vi "Sub Super Duper_7_02a_JW.vi"(0 "VISA resource name":refnum<visa-resource-name>="GPIB0::17::INSTR", 1 "Sample Properties:":T5 {"Date Created" format="%<%Y/%m/%d>T"}, 2 "TRF Cluster":T6={"Step 4"=-38.0, "# of Loops"=1.0, "Transfer 2"=FALSE, "Start 4"=-2.0, "Total Points 2"=2, "Start 3"=40.0, "Stop 2"=-40.0, "Step 3"=-1.0, "Loop Step"=0.0, "Integration Time 3"=0, "Loop Wait"=0.0, "First Step"=0.0} {"Loop Wait" format="%<%H:%M:%S>t"; "Integration Time 3" scale=0.0..2.0; "Step 3" format="%.2f"; "Stop 2" format="%.2f"; "Start 3" format="%.2f"; "Start 4" format="%.2f"; "Step 4" format="%.2f"}, 3 "TSP Cluster":T7={"Transport"=FALSE, "Start 2"=0.0, "Stop 3"=-60.0, "Step 2"=-1.0, "Start"=0.0, "Step"=-10.0, "Total Points"=7, "Integration Time"=0} {"Integration Time" scale=0.0..2.0; "Step" format="%.2f"; "Start" format="%.2f"; "Step 2" format="%.2f"; "Stop 3" format="%.2f"; "Start 2" format="%.2f"}, 4 "Compliance Cluster":T2={"Var1 sweep settings"={"sweep spacing (linear: 0)"=0, "sweep mode"=FALSE, "compliance (V)"=100.0, "compliance (A)"=0.001}, "Var1 sweep settings 2"={"sweep spacing (linear: 0)"=0, "sweep mode"=FALSE, "compliance (V)"=100.0, "compliance (A)"=0.001}, "Var2 step settings 2"={"compliance (A)"=0.001, "compliance (V)"=100.0}, "Var2 step settings"={"compliance (A)"=0.001, "compliance (V)"=100.0}} {"Var2 step settings"."compliance (V)" format="%.2f"; "Var2 step settings"."compliance (A)" format="%^.2e"; "Var2 step settings 2"."compliance (V)" format="%.2f"; "Var2 step settings 2"."compliance (A)" format="%^.2e"; "Var1 sweep settings 2"."compliance (A)" format="%^.2e"; "Var1 sweep settings 2"."compliance (V)" format="%.2f"; "Var1 sweep settings 2"."sweep spacing (linear: 0)" items=["linear", "log 10", "log 25", "log 50"]; "Var1 sweep settings"."compliance (A)" format="%^.2e"; "Var1 sweep settings"."compliance (V)" format="%.2f"; "Var1 sweep settings"."sweep spacing (linear: 0)" items=["linear", "log 10", "log 25", "log 50"]}, 5 "error in":errorcluster, 6 "Saved Folder:":path=path "C:/1DATA/2011", 7 "Wait Cluster":T1 {"Wait Time (s)" format="%.1g"; "Wait Countdown" format="%<%H:%M:%S%1u>t"}, 9 "Stop \nCountdown":bool) -> (8 "Status Indicator":bool, 14 "VISA resource name out":refnum<visa-resource-name>, 15 "TRF Path":path, 16 "TSP Path":path, 17 "Graph Cluster":T3, 18 "Char Cluster":T4, 19 "error out":errorcluster)   [LabVIEW 2011]
uses:
  <vilib>/Platform/TimedLoop/XDataNode/timing_clust.ctl
  <vilib>/Platform/TimedLoop/XDataNode/nitl_modes.ctl
  <vilib>/Platform/TimedLoop/XDataNode/wakeup.ctl
  <vilib>/Platform/TimedLoop/XDataNode/XDataNode.xnode
  <vilib>/Platform/TimedLoop/XDataNode/XDNodeRunTimeDep.lvlib
panel:
  in  "Transport Temp":cluster{"trace":dbl[], "trace":dbl[]}(graph)
  in  "Transfer Temp":cluster{dbl[], "trace":dbl[]}[](graph) caption="Transfer"
  # "Vg Sweep"
  # "Vd Step"
  # "Loops and Integration Time"
  # "Device Characteristics"
  # "Sample Properties:"
  # "%"
  # "nm"
  # "Device Properties:"
  # "um"
  # "um"
  # "Vg Step"
  # "Vd Step"
  # "Integration Time"
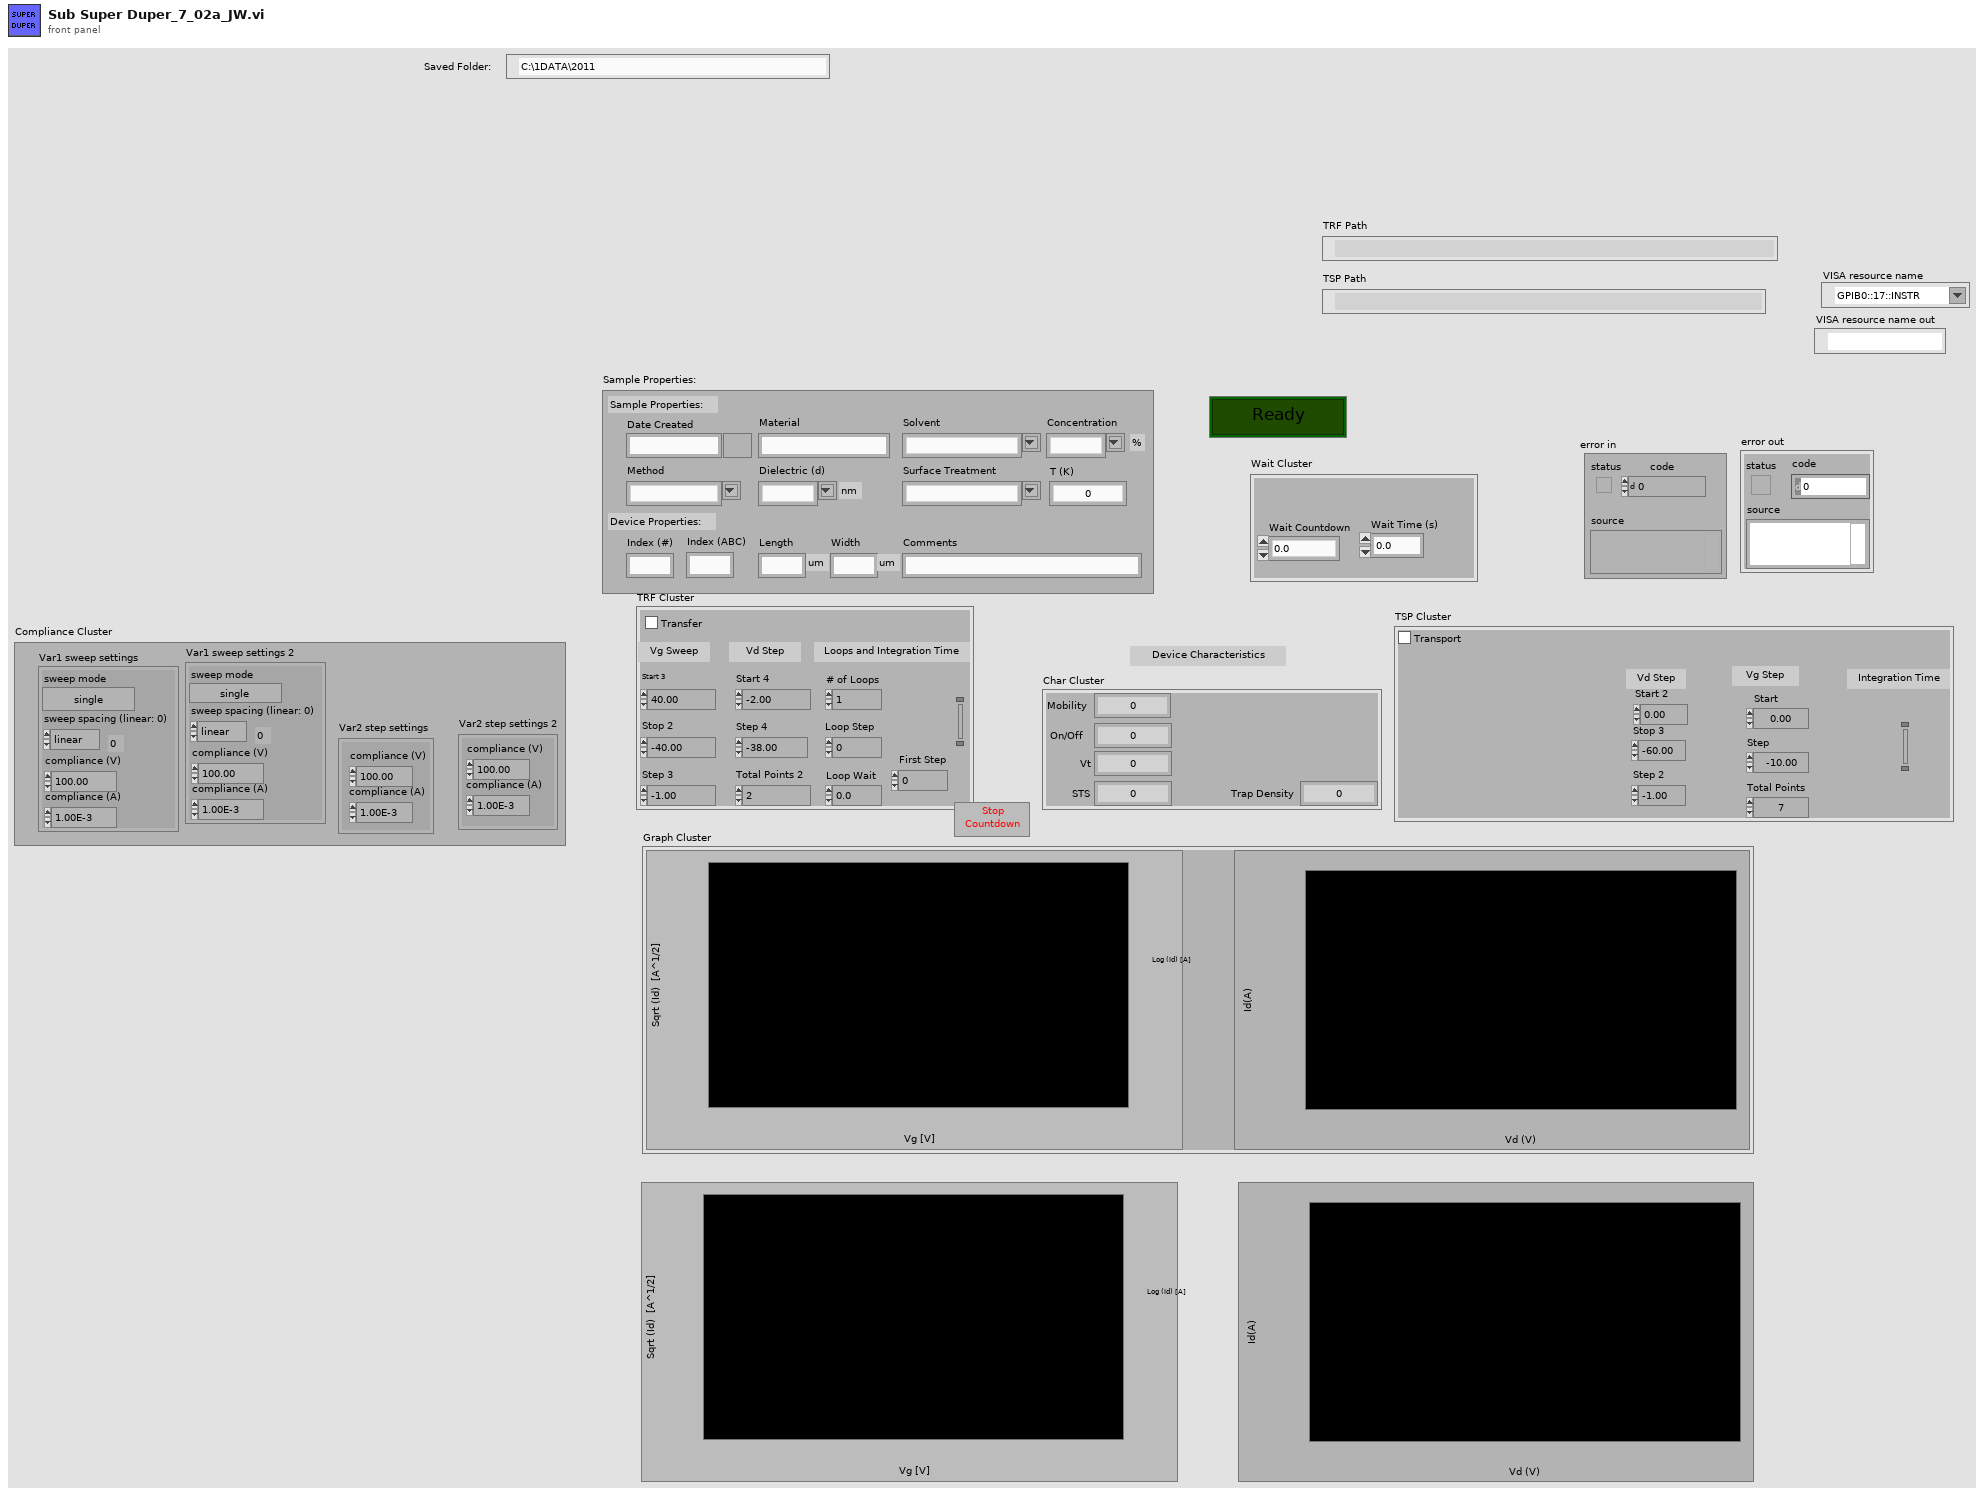
[diagram p1: front panel]
types:
  T1 = cluster{"Wait Countdown":dbl, "Wait Time (s)":dbl}
  T2 = cluster{"Var1 sweep settings":cluster{"sweep spacing (linear: 0)":u16, "sweep mode":bool, "compliance (V)":dbl, "compliance (A)":dbl}, "Var1 sweep settings 2":cluster{"sweep spacing (linear: 0)":u16, "sweep mode":bool, "compliance (V)":dbl, "compliance (A)":dbl}, "Var2 step settings 2":cluster{"compliance (A)":dbl, "compliance (V)":dbl}, "Var2 step settings":cluster{"compliance (A)":dbl, "compliance (V)":dbl}}
  T3 = cluster{"Transfer":cluster{dbl[], "trace":dbl[]}[], "Transport":cluster{"trace":dbl[], "trace":dbl[]}}
  T4 = cluster{"Mobility":dbl, "On/Off ":dbl, "Vt":dbl, "STS":dbl, "Trap Density":dbl}
  T5 = cluster{"Date Created":timestamp, "Material":string, "Solvent":string, "Concentration":string, "Method":string, "Dielectric (d)":string, "Index (#)":string, "Index (ABC)":string, "Length":string, "Width":string, "Surface Treatment":string, "Comments":string, "T (K)":dbl}
  T6 = cluster{"Step 4":dbl, "# of Loops":dbl, "Transfer 2":bool, "Start 4":dbl, "Total Points 2":u16, "Start 3":dbl, "Stop 2":dbl, "Step 3":dbl, "Loop Step":dbl, "Integration Time 3":u32, "Loop Wait":dbl, "First Step":dbl}
  T7 = cluster{"Transport":bool, "Start 2":dbl, "Stop 3":dbl, "Step 2":dbl, "Start":dbl, "Step":dbl, "Total Points":u16, "Integration Time":u32}
  T8 = typedef "XDNodeRunTimeDep.lvlib/timing_clust.ctl" = cluster{"Expected End [f-1]":u64, "Actual End [f-1]":u64, "Finished Late? [f-1]":bool, "Expected End [i-1]":u64, "Actual End [i-1]":u64, "Finished Late? [i-1]":bool, "Expected Start [i]":u64, "Actual Start [i]":u64, "Expected Start [f]":u64, "Actual Start [f]":u64, "Source Name":string, "Structure Name":string, "Period":i64, "Deadline":i64, "Offset":i64, "Start":i64, "Priority":i32, "Timeout":i32, "Mode":T9, "Wakeup Reason":T10, "Error":errorcluster, "Source Type":string, "Secondary Source Type":string, "Global End Time":u64, "Global Start Time":u64, "Frame Duration":u64, "Iteration Duration":u64, "Assigned CPU":i32, "I/O Scan Engine Mode":u32}
  T9 = typedef "XDNodeRunTimeDep.lvlib/nitl_modes.ctl" = enum32{"No Change", "Process missed periods, maintain original phase", "Discard missed periods, maintain original phase", "Process missed periods, ignore original phase", "Discard missed periods, ignore original phase"}
  T10 = typedef "XDNodeRunTimeDep.lvlib/wakeup.ctl" = enum32{"Normal", "Aborted", "Asynchronous wakeup", "Timing source error", "Timed loop error", "Timeout"}
  T11 = cluster{"sweep spacing (linear: 0)":u16, "sweep mode":bool, "compliance (V)":dbl, "compliance (A)":dbl}
  T12 = cluster{"compliance (A)":dbl, "compliance (V)":dbl}
  T13 = cluster{"Start 3":dbl, "Stop 2":dbl, "Step 3":dbl, "sweep spacing (linear: 0)":u16, "sweep mode":bool, "compliance (V)":dbl, "compliance (A)":dbl}
  T14 = cluster{"compliance (A)":dbl, "compliance (V)":dbl, "Start 4":dbl, "Total Points 2":u16, dbl}
  T15 = cluster{"Mobility":dbl, "On/Off Current":dbl, "Vt":dbl, "STS":dbl, "Trap Density":dbl}
  T16 = cluster{"Start 2":dbl, "Stop 3":dbl, "Step 2":dbl, "sweep spacing (linear: 0)":u16, "sweep mode":bool, "compliance (V)":dbl, "compliance (A)":dbl}
  T17 = cluster{"compliance (A)":dbl, "compliance (V)":dbl, "Start":dbl, "Total Points":u16, "Step":dbl}
  T18 = cluster{"Transfer Temp":cluster{dbl[], "trace":dbl[]}[], "Transport Temp":cluster{"trace":dbl[], "trace":dbl[]}}
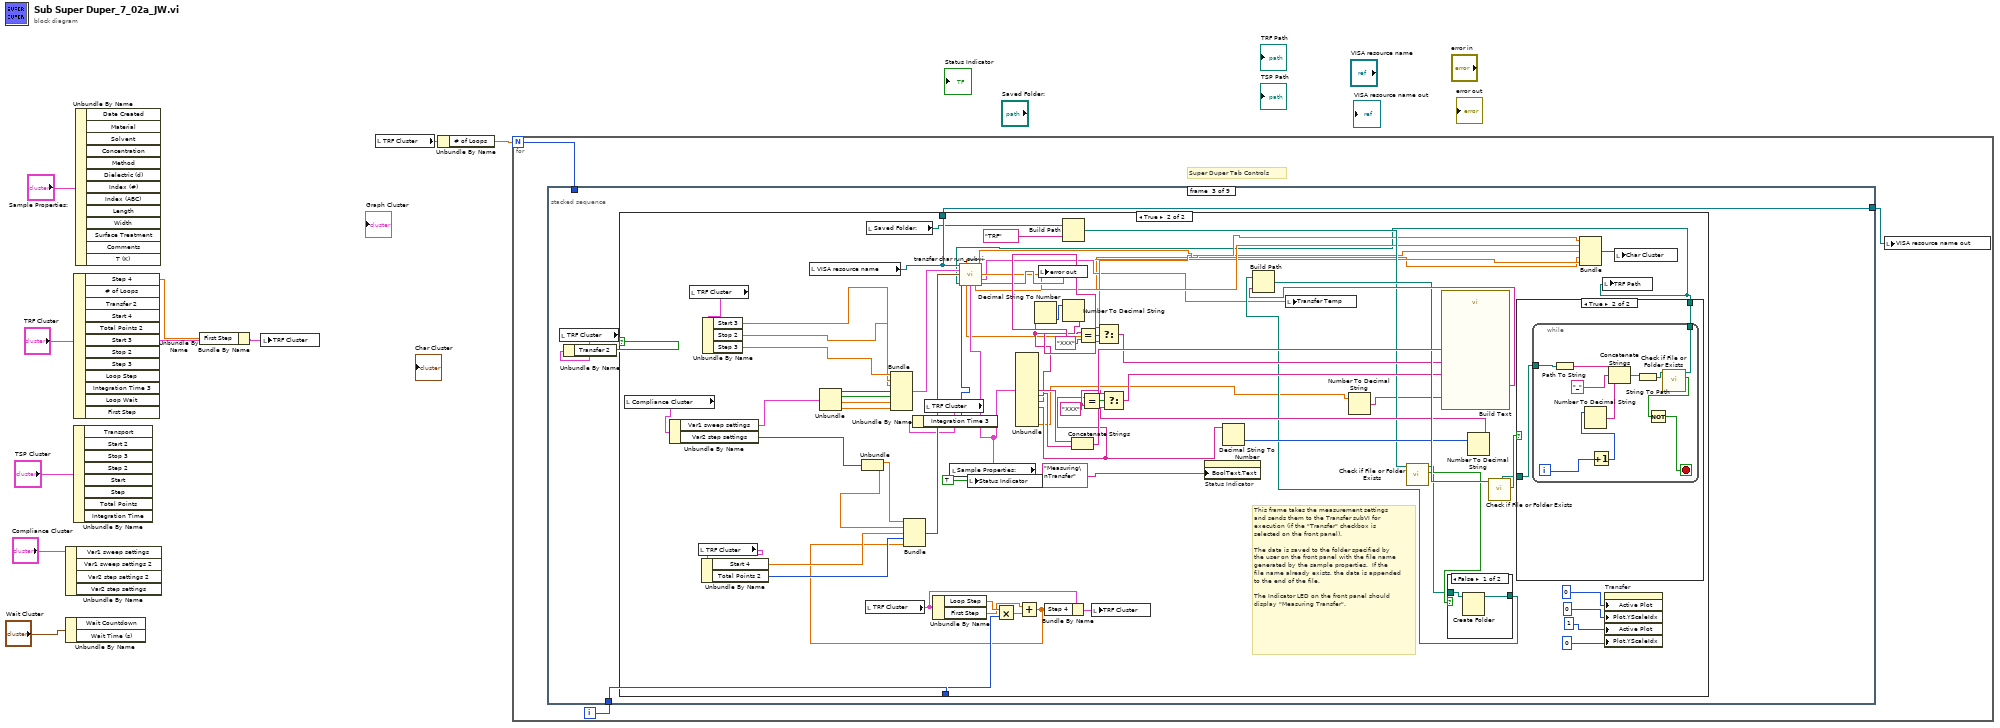
[diagram p0: block diagram]
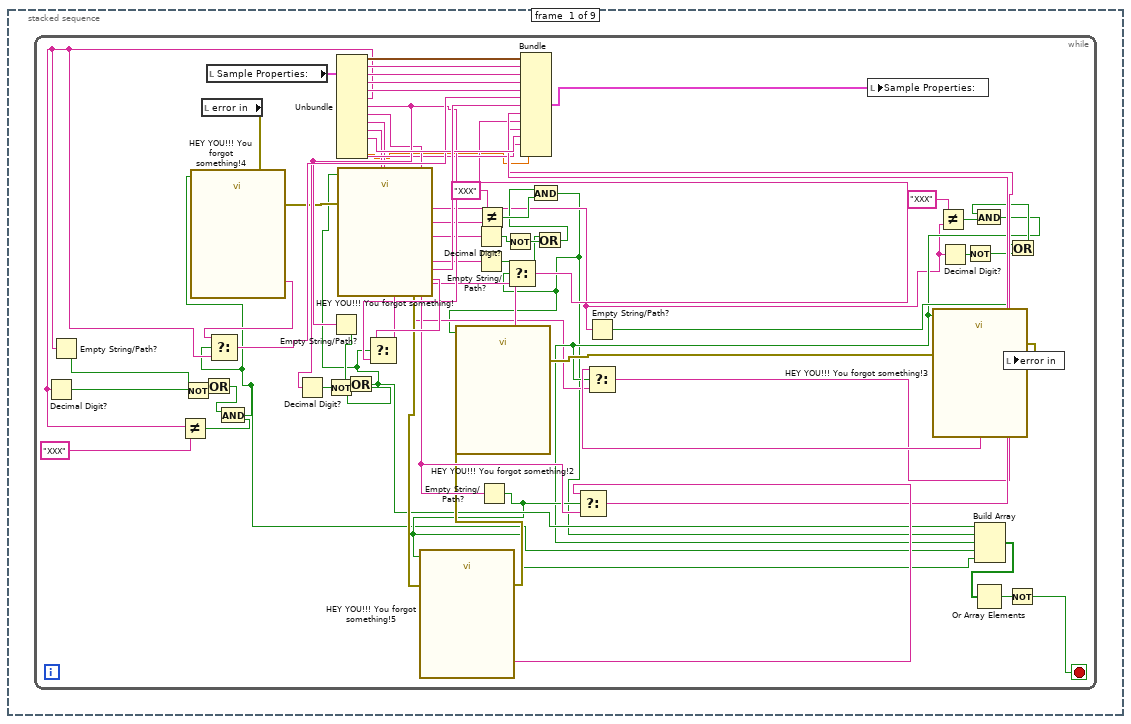
[diagram p2: hidden frame]
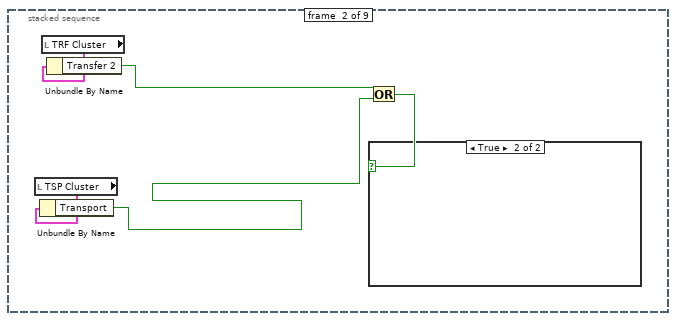
[diagram p3: hidden frame]
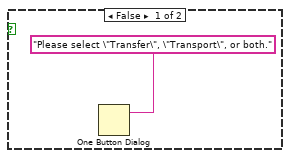
[diagram p4: hidden frame]
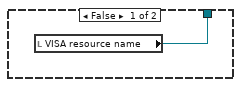
[diagram p5: hidden frame]
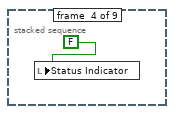
[diagram p8: hidden frame]
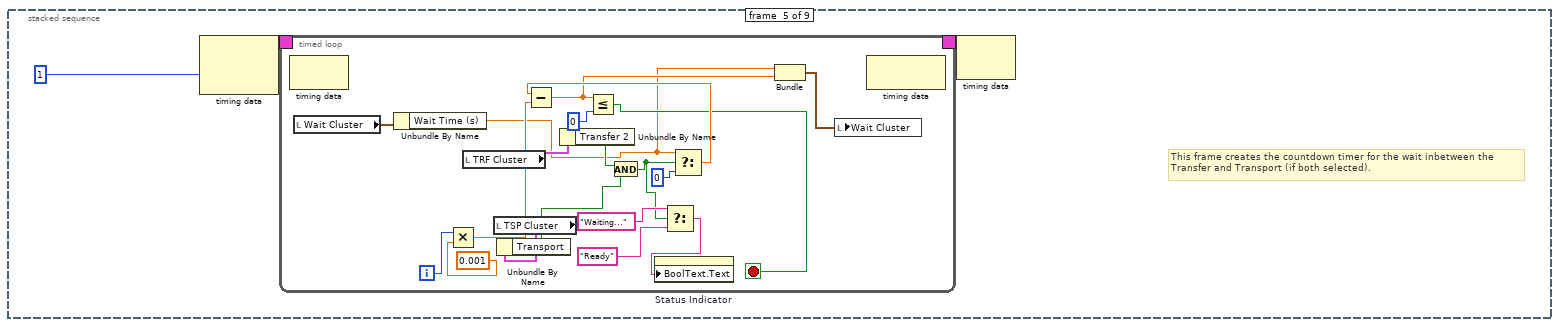
[diagram p9: hidden frame]
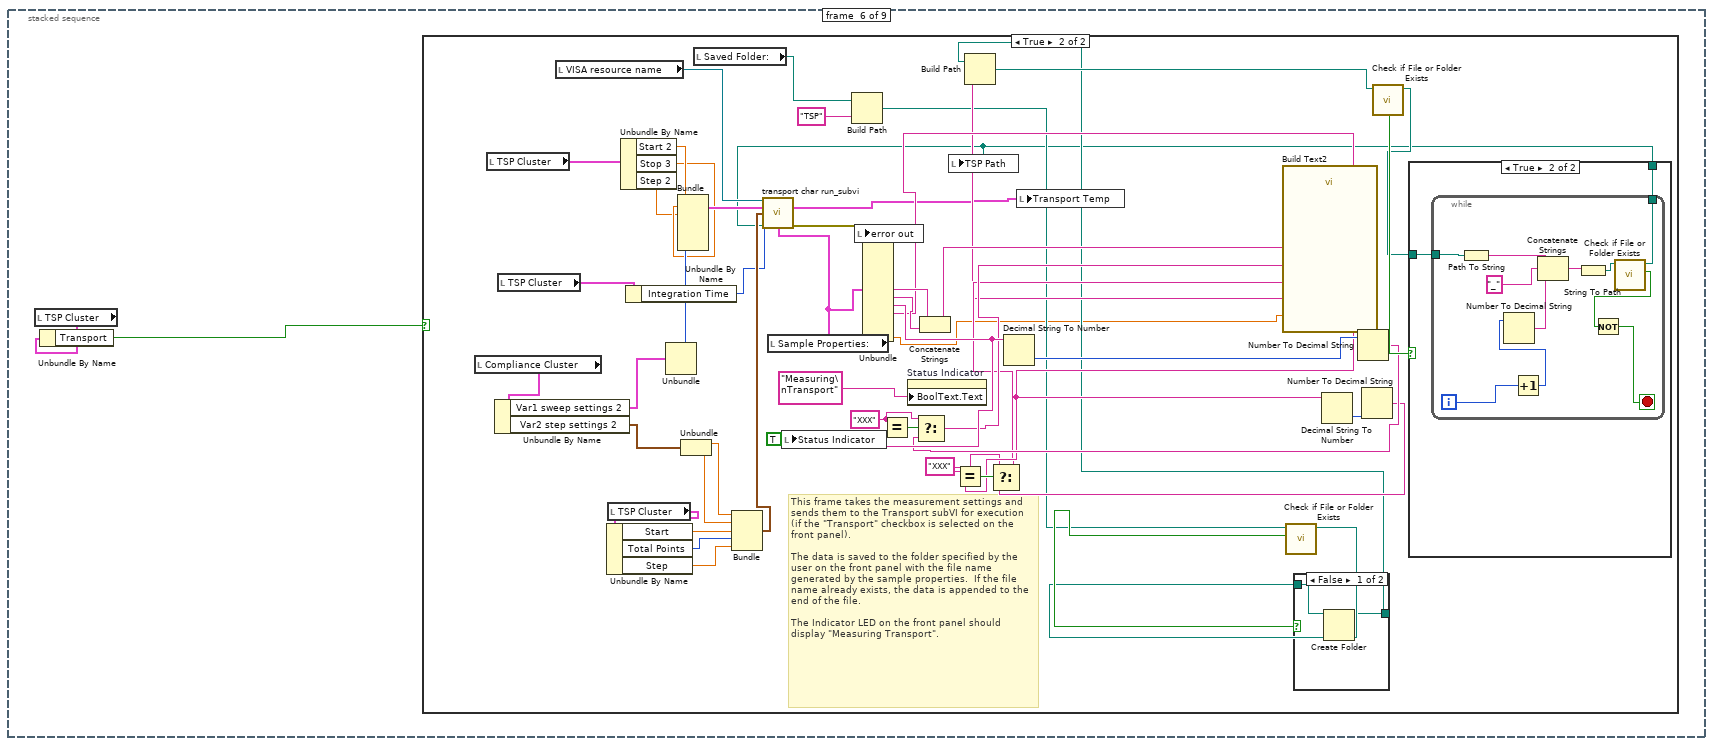
[diagram p10: hidden frame]
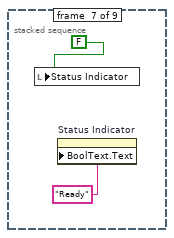
[diagram p14: hidden frame]
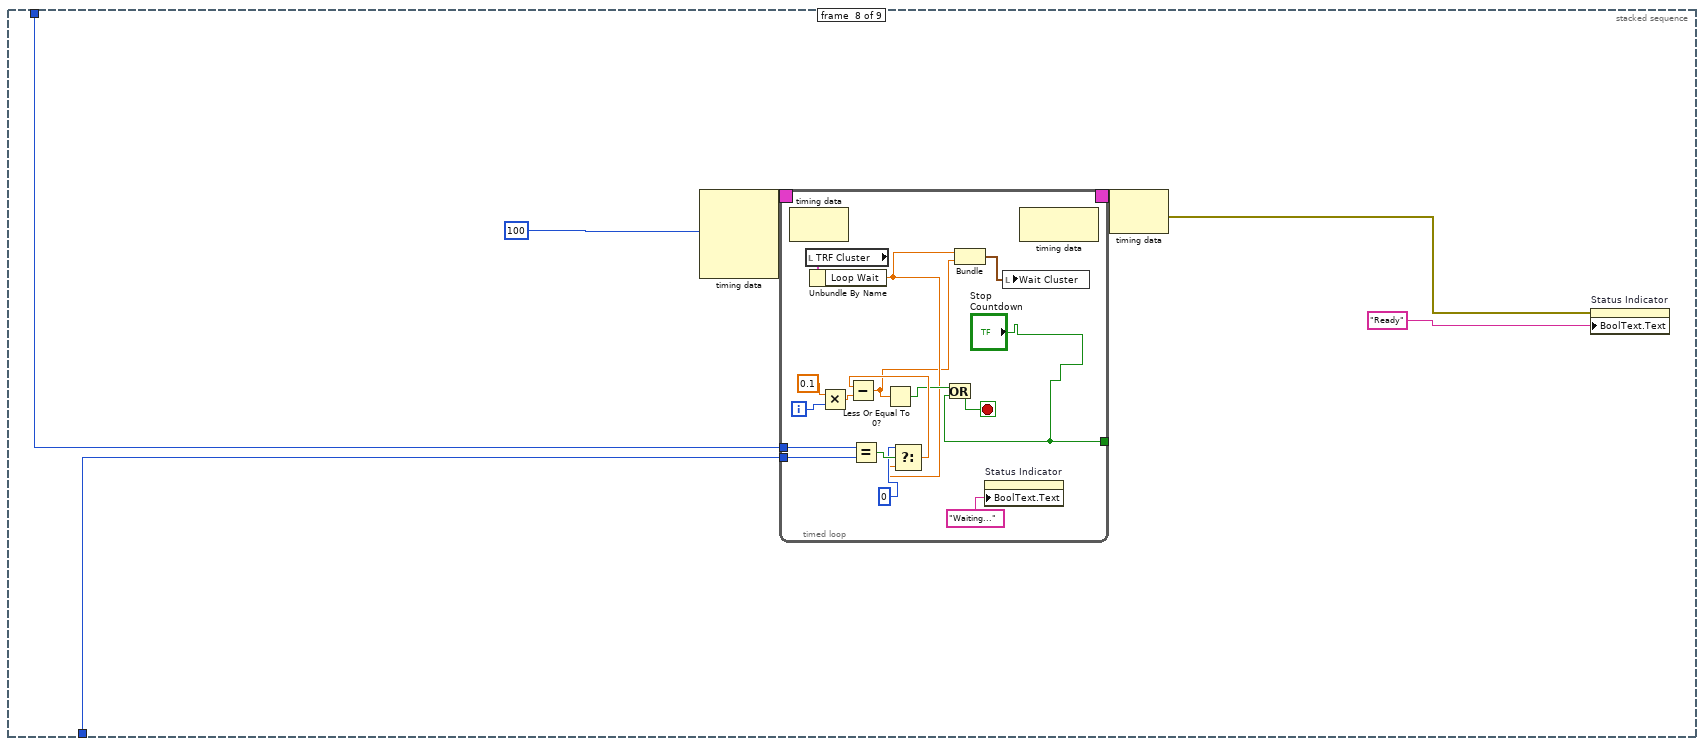
[diagram p15: hidden frame]
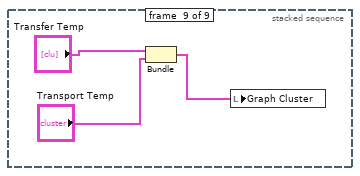
[diagram p16: hidden frame]
diagram:
  n1 = Unbundle By Name("Compliance Cluster") -> ()  [unwired: 4 out]
  n2 = Unbundle By Name("Wait Cluster") -> ()  [unwired: 2 out]
  n3 = Unbundle By Name("TSP Cluster") -> ()  [unwired: 8 out]
  n4 = Unbundle By Name("TRF Cluster") -> ("Step 4"=w1:dbl)  [unwired: 11 out]
  n5 = Unbundle By Name("Sample Properties:") -> ()  [unwired: 13 out]
  n6 = Bundle By Name(cluster="TRF Cluster", "First Step"=w1) -> (w3:T6)
  n7 = local write "TRF Cluster"(w3) -> ()
  n8 = local read "TRF Cluster"() -> (w9:T6)
  n9 = Unbundle By Name(w9) -> ("# of Loops"=w8:dbl)
  n10 = for {
    N: w8 -> [w11]
    i -> [w12]
    # "Super Duper Tab Controls"
    n11 = stacked-sequence {
      tunnel: w12 -> [_ _ w82 _ _ _ _ w277 _]
      tunnel: w11 -> [_ _ _ _ _ _ _ w276 _]
      tunnel: [_ _ w79 _ _ _ _ _ _] -> w10
      frame #0 {
        n12 = while {
          stop <- w38 stop-if-true
          n13 = local read "error in"() -> (w44:errorcluster)
          n14 = local read "Sample Properties:"() -> (w67:T5)
          n15 = Unbundle(w67) -> ("Date Created"=w68:timestamp, "Material"=w69:string, "Solvent"=w70:string, "Concentration"=w71:string, "Method"=w72:string, "Dielectric (d)"=w27:string, "Index (#)"=w57:string, "Index (ABC)"=w54:string, "Length"=w22:string, "Width"=w15:string, "Surface Treatment"=w60:string, "Comments"=w52:string, "T (K)"=w13:dbl)
          n16 = Decimal Digit?(1:w27) -> (0:w35:bool)
          n17 = Empty String/Path?(string/path=w27) -> (empty?=w29:bool)
          n18 = Not Equal?(x=w27, y="XXX") -> (x != y?=w26:bool)
          n19 = Not(x=w35) -> (.not. x?=w32:bool)
          n20 = Or(x=w29, y=w32) -> (x .or. y?=w25:bool)
          n21 = And(x=w25, y=w26) -> (x .and. y?=w24:bool)
          n22 = call "HEY YOU!!! You forgot something!4"("Enable"=w24, "error in (no error)"=w44) -> ("Dielectric (d)"=w59:string, "error out"=w43:errorcluster)  [unwired: 15 in, 1 out]
          n23 = Select(t=w59, s=w24, f=w27) -> (s? t:f=w58:string)
          n24 = Decimal Digit?(1:w57) -> (0:w48:bool)
          n25 = Not(x=w48) -> (.not. x?=w47:bool)
          n26 = Empty String/Path?(string/path=w57) -> (empty?=w56:bool)
          n27 = Or(x=w56, y=w47) -> (x .or. y?=w42:bool)
          n28 = call "HEY YOU!!! You forgot something!"("Enable"=w42, "error in (no error)"=w43) -> ("Index (#)"=w66:string, "error out"=w46:errorcluster)  [unwired: 15 in, 1 out]
          n29 = Select(t=w66, s=w42, f=w57) -> (s? t:f=w63:string)
          n30 = Decimal Digit?(1:w22) -> (0:w37:bool)
          n31 = Empty String/Path?(string/path=w22) -> (empty?=w31:bool)
          n32 = Not Equal?(x="XXX", y=w22) -> (x != y?=w21:bool)
          n33 = Empty String/Path?(string/path=w54) -> (empty?=w41:bool)
          n34 = call "HEY YOU!!! You forgot something!5"("Enable"=w41, "error in (no error)"=w46) -> ("Index (ABC)"=w55:string, "error out"=w45:errorcluster)  [unwired: 15 in, 1 out]
          n35 = Not(x=w37) -> (.not. x?=w34:bool)
          n36 = Or(x=w31, y=w34) -> (x .or. y?=w20:bool)
          n37 = And(x=w20, y=w21) -> (x .and. y?=w14:bool)
          n38 = call "HEY YOU!!! You forgot something!2"("Enable"=w14, "error in (no error)"=w45) -> ("Length"=w65:string, "error out"=w62:errorcluster)  [unwired: 15 in, 1 out]
          n39 = Select(t=w65, s=w14, f=w22) -> (s? t:f=w51:string)
          n40 = Select(t=w55, s=w41, f=w54) -> (s? t:f=w53:string)
          n41 = Empty String/Path?(string/path=w15) -> (empty?=w30:bool)
          n42 = Not Equal?(x="XXX", y=w15) -> (x != y?=w19:bool)
          n43 = Decimal Digit?(1:w15) -> (0:w36:bool)
          n44 = Not(x=w36) -> (.not. x?=w33:bool)
          n45 = Or(x=w30, y=w33) -> (x .or. y?=w18:bool)
          n46 = And(x=w18, y=w19) -> (x .and. y?=w17:bool)
          n47 = call "HEY YOU!!! You forgot something!3"("Enable"=w17, "error in (no error)"=w62) -> ("Width"=w64:string, "error out"=w61:errorcluster)  [unwired: 15 in, 1 out]
          n48 = Select(t=w64, s=w17, f=w15) -> (s? t:f=w50:string)
          n49 = Bundle("Date Created"=w68, "Material"=w69, "Solvent"=w70, "Concentration"=w71, "Method"=w72, "Dielectric (d)"=w58, "Index (#)"=w63, "Index (ABC)"=w53, "Length"=w51, "Width"=w50, "Surface Treatment"=w60, "Comments"=w52, "T (K)"=w13) -> (w49:T5)  [unwired: 1 in]
          n50 = local write "Sample Properties:"(w49) -> ()
          n51 = Build Array(w42, w14, w17, w24, w41) -> (w40:bool[])
          n52 = Or Array Elements(Boolean array=w40) -> (logical OR=w39:bool)
          n53 = local write "error in"(w61) -> ()
          n54 = Not(x=w39) -> (.not. x?=w38:bool)
        }
      }
      frame #1 {
        n55 = local read "TSP Cluster"() -> (w74:T7)
        n56 = Unbundle By Name(w74) -> ("Transport"=w73:bool)
        n57 = local read "TRF Cluster"() -> (w76:T6)
        n58 = Unbundle By Name(w76) -> ("Transfer 2"=w75:bool)
        n59 = Or(x=w75, y=w73) -> (x .or. y?=w77:bool)
        n60 = case shown="True" w77 {
          frame False {
            n61 = One Button Dialog(message="Please select \"Transfer\", \"Transport\", or both.") -> ()  [unwired: 1 in, 1 out]
          }
          frame True {
          }
        }
      }
      frame #2 {
        n62 = local read "TRF Cluster"() -> (w80:T6)
        n63 = Unbundle By Name(w80) -> ("Transfer 2"=w81:bool)
        n64 = case shown="True" w81 {
          tunnel: w82 -> [_ w91]
          tunnel: [w83 w100] -> w79
          frame False {
            n65 = local read "VISA resource name"() -> (w83:refnum<visa-resource-name>)
          }
          frame True {
            w130 = "XXX"
            w134 = "XXX"
            # "This frame takes the measurement settings and sends them to the Transfer subVI for execution (if the \"Transfer\" checkbox is selected on the front panel).\n\nThe data is saved to the folder specified by the user on the front panel with the file name generated by the sample properties.  If the file name already exists, the data is appended to the end of the file.\n\nThe Indicator LED on the front panel should display \"Measuring Transfer\"."
            n66 = local read "Compliance Cluster"() -> (w97:T2)
            n67 = Unbundle By Name(w97) -> ("Var1 sweep settings"=w95:T11, "Var2 step settings"=w96:T12)
            n68 = local read "TRF Cluster"() -> (w111:T6)
            n69 = local read "TRF Cluster"() -> (w114:T6)
            n70 = Unbundle By Name(w114) -> ("Start 4"=w113:dbl, "Total Points 2"=w112:u16)
            n71 = Unbundle By Name(w111) -> ("Start 3"=w110:dbl, "Stop 2"=w109:dbl, "Step 3"=w108:dbl)
            n72 = local read "VISA resource name"() -> (w100:refnum<visa-resource-name>)
            n73 = Unbundle(w95) -> ("sweep spacing (linear: 0)"=w154:u16, "sweep mode"=w153:bool, "compliance (V)"=w152:dbl, "compliance (A)"=w151:dbl)
            n74 = Unbundle(w96) -> ("compliance (A)"=w149:dbl, "compliance (V)"=w148:dbl)
            n75 = local read "TRF Cluster"() -> (w86:T6)
            n76 = local read "Saved Folder:"() -> (w99:path)
            n77 = Bundle("Start 3"=w110, "Stop 2"=w109, "Step 3"=w108, "sweep spacing (linear: 0)"=w154, "sweep mode"=w153, "compliance (V)"=w152, "compliance (A)"=w151) -> (w150:T13)  [unwired: 1 in]
            n78 = local read "TRF Cluster"() -> (w106:T6)
            n79 = Unbundle By Name(w106) -> ("Integration Time 3"=w107:u32)
            n80 = Unbundle By Name(w86) -> ("Loop Step"=w89:dbl, "First Step"=w88:dbl)
            n81 = local read "Sample Properties:"() -> (w116:T5)
            n82 = local write "Status Indicator"(TRUE) -> ()
            n83 = Multiply(x=w89, y=w91) -> (x*y=w92:dbl)
            n84 = Unbundle(w116) -> ("Index (#)"=w143:string, "Index (ABC)"=w142:string, "Length"=w126:string, "Width"=w129:string, "T (K)"=w94:dbl)  [unwired: 8 out]
            n85 = Add(x=w88, y=w92) -> (x+y=w87:dbl)
            n86 = Bundle("compliance (A)"=w149, "compliance (V)"=w148, "Start 4"=w113, "Total Points 2"=w112, w87) -> (w147:T14)  [unwired: 1 in]
            n87 = Decimal String To Number(string=w126) -> (number=w137:i32)  [unwired: 2 in, 1 out]
            n88 = Bundle By Name(cluster=w86, "Step 4"=w87) -> (w90:T6)
            n89 = Build Path(base path=w99, name or relative path="TRF") -> (appended path=w122:path)
            n90 = Number To Decimal String(number=w137) -> (decimal integer string=w133:string)  [unwired: 1 in]
            n91 = Concatenate Strings(w143, w142) -> (w141:string)
            n92 = Equal?(x=w126, y=w134) -> (x = y?=w135:bool)
            n93 = Equal?(x=w129, y=w130) -> (x = y?=w131:bool)
            n94 = local write "TRF Cluster"(w90) -> ()
            n95 = Select(t=w134, s=w135, f=w133) -> (s? t:f=w132:string)
            n96 = property on="Status Indicator" class="Bool (strict)"("BoolText.Text"="Measuring\nTransfer") -> ()  [unwired: 2 in, 2 out]
            n97 = Decimal String To Number(string=w129) -> (number=w136:i32)  [unwired: 2 in, 1 out]
            n98 = Number To Decimal String(number=w94) -> (decimal integer string=w93:string)  [unwired: 1 in]
            n99 = call <vilib>:"Check if File or Folder Exists.vi"("path"=w122) -> ("file or folder exists?"=w124:bool, "dup path"=w123:path)  [unwired: 8 in, 1 out]
            n100 = case shown="False" w124 {
              tunnel: w123 -> [w156 w157]
              tunnel: [w155 w157] -> w121
              frame False {
                n101 = Create Folder(path (use dialog)=w156) -> (created path=w155:path)  [unwired: 2 in, 2 out]
              }
              frame True {
              }
            }
            n102 = Number To Decimal String(number=w136) -> (decimal integer string=w128:string)  [unwired: 1 in]
            n103 = Select(t=w130, s=w131, f=w128) -> (s? t:f=w127:string)
            n104 = call "Build Text"("T"=w93, "Index"=w141, "Length"=w132, "Width"=w127) -> ("Result"=w146:string)  [unwired: 10 in, 1 out]
            n105 = Build Path(base path=w121, name or relative path=w146) -> (appended path=w139:path)
            n106 = call <vilib>:"Check if File or Folder Exists.vi"("path"=w139) -> ("file or folder exists?"=w140:bool, "dup path"=w138:path)  [unwired: 8 in, 1 out]
            n107 = case shown="True" w140 {
              tunnel: w138 -> [w158 w160]
              tunnel: [w158 w159] -> w98
              frame False {
              }
              frame True {
                n108 = while {
                  tunnel: w160 -> [w162]
                  tunnel: [w161] -> w159
                  i -> [w164]
                  stop <- w165 stop-if-true
                  n109 = Path To String(path=w162) -> (string=w171:string)
                  n110 = Increment(x=w164) -> (x+1=w163:i32)
                  n111 = Number To Decimal String(number=w163) -> (decimal integer string=w169:string)  [unwired: 1 in]
                  n112 = Concatenate Strings(w171, "_", w169) -> (w168:string)
                  n113 = String To Path(string=w168) -> (path=w167:path)
                  n114 = call <vilib>:"Check if File or Folder Exists.vi"("path"=w167) -> ("file or folder exists?"=w166:bool, "dup path"=w161:path)  [unwired: 8 in, 1 out]
                  n115 = Not(x=w166) -> (.not. x?=w165:bool)
                }
              }
            }
            n116 = call "transfer char run_subvi.vi"("VISA session"=w100, "Var1 sweep settings"=w150, "Var2 step settings"=w147, "integration time"=w107, "Path"=w98, "Sample Properties:"=w116) -> ("Trap Density"=w85:dbl, "Mobility"=w104:dbl, "On/Off Current"=w103:dbl, "XY Graph"=w101:cluster{dbl[], "trace":dbl[]}[], "Vt"=w102:dbl, "STS"=w84:dbl, "error?"=w115:errorcluster)  [unwired: 2 in, 1 out]
            n117 = local write "error out"(w115) -> ()
            n118 = local write "Transfer Temp"(w101) -> ()
            n119 = Bundle("Mobility"=w104, "On/Off Current"=w103, "Vt"=w102, "STS"=w84, "Trap Density"=w85) -> (w105:T15)  [unwired: 1 in]
            n120 = local write "TRF Path"(w98) -> ()
            n121 = property on="Transfer" class="XYGraph (strict)"("Active Plot"=0, "Plot.YScaleIdx"=0, "Active Plot"=1, "Plot.YScaleIdx"=0) -> ()  [unwired: 2 in, 2 out]
            n122 = local write "Char Cluster"(w105) -> ()
          }
        }
      }
      frame #3 {
        n123 = local write "Status Indicator"(FALSE) -> ()
      }
      frame #4 {
        # "This frame creates the countdown timer for the wait inbetween the\nTransfer and Transport (if both selected)."
        n124 = node-c288(1) -> (w175:T8)  [unwired: 1 in]
        n125 = timed-loop {
          timing: w175 -> [_]
          timing-out: [_] -> w174
          i -> [w186]
          stop <- w187 stop-if-true
          n126 = node-c288() -> ()  [unwired: 1 in, 1 out]
          n127 = local read "Wait Cluster"() -> (w179:T1)
          n128 = Unbundle By Name(w179) -> ("Wait Time (s)"=w177:dbl)
          n129 = Multiply(x=w186, y=0.001) -> (x*y=w184:dbl)
          n130 = local read "TRF Cluster"() -> (w180:T6)
          n131 = local read "TSP Cluster"() -> (w181:T7)
          n132 = Unbundle By Name(w181) -> ("Transport"=w182:bool)
          n133 = Unbundle By Name(w180) -> ("Transfer 2"=w183:bool)
          n134 = And(x=w183, y=w182) -> (x .and. y?=w191:bool)
          n135 = Select(t="Waiting...", s=w191, f="Ready") -> (s? t:f=w193:string)
          n136 = property on="Status Indicator" class="Bool (strict)"("BoolText.Text"=w193) -> ()  [unwired: 2 in, 2 out]
          n137 = Select(t=w177, s=w191, f=0) -> (s? t:f=w189:dbl)
          n138 = Subtract(x=w189, y=w184) -> (x-y=w178:dbl)
          n139 = Less Or Equal?(x=w178, y=0) -> (x <= y?=w187:bool)
          n140 = Bundle("Wait Time (s)"=w177, w178) -> (w176:cluster{"Wait Time (s)":dbl, dbl})  [unwired: 1 in]
          n141 = local write "Wait Cluster"(w176) -> ()
          n142 = node-c288() -> ()  [unwired: 1 in, 1 out]
        }
        n143 = node-c288(w174) -> ()  [unwired: 1 out]
      }
      frame #5 {
        n144 = local read "TSP Cluster"() -> (w202:T7)
        n145 = Unbundle By Name(w202) -> ("Transport"=w201:bool)
        n146 = case shown="True" w201 {
          frame False {
          }
          frame True {
            w229 = "XXX"
            w233 = "XXX"
            # "This frame takes the measurement settings and sends them to the Transport subVI for execution (if the \"Transport\" checkbox is selected on the front panel).\n\nThe data is saved to the folder specified by the user on the front panel with the file name generated by the sample properties.  If the file name already exists, the data is appended to the end of the file.\n\nThe Indicator LED on the front panel should display \"Measuring Transport\"."
            n147 = local read "Compliance Cluster"() -> (w207:T2)
            n148 = local read "TSP Cluster"() -> (w220:T7)
            n149 = Unbundle By Name(w207) -> ("Var1 sweep settings 2"=w206:T11, "Var2 step settings 2"=w205:T12)
            n150 = local read "TSP Cluster"() -> (w213:T7)
            n151 = local read "VISA resource name"() -> (w209:refnum<visa-resource-name>)
            n152 = local read "TSP Cluster"() -> (w211:T7)
            n153 = Unbundle By Name(w211) -> ("Start"=w216:dbl, "Total Points"=w215:u16, "Step"=w214:dbl)
            n154 = Unbundle By Name(w220) -> ("Start 2"=w219:dbl, "Stop 3"=w218:dbl, "Step 2"=w217:dbl)
            n155 = Unbundle By Name(w213) -> ("Integration Time"=w212:u32)
            n156 = Unbundle(w206) -> ("sweep spacing (linear: 0)"=w256:u16, "sweep mode"=w255:bool, "compliance (V)"=w254:dbl, "compliance (A)"=w253:dbl)
            n157 = Bundle("Start 2"=w219, "Stop 3"=w218, "Step 2"=w217, "sweep spacing (linear: 0)"=w256, "sweep mode"=w255, "compliance (V)"=w254, "compliance (A)"=w253) -> (w252:T16)  [unwired: 1 in]
            n158 = Unbundle(w205) -> ("compliance (A)"=w251:dbl, "compliance (V)"=w250:dbl)
            n159 = local read "Saved Folder:"() -> (w208:path)
            n160 = Bundle("compliance (A)"=w251, "compliance (V)"=w250, "Start"=w216, "Total Points"=w215, "Step"=w214) -> (w249:T17)  [unwired: 1 in]
            n161 = local read "Sample Properties:"() -> (w245:T5)
            n162 = local write "Status Indicator"(TRUE) -> ()
            n163 = Build Path(base path=w208, name or relative path="TSP") -> (appended path=w222:path)
            n164 = Unbundle(w245) -> ("Index (#)"=w244:string, "Index (ABC)"=w243:string, "Length"=w234:string, "Width"=w230:string, "T (K)"=w203:dbl)  [unwired: 8 out]
            n165 = Equal?(x=w233, y=w234) -> (x = y?=w235:bool)
            n166 = property on="Status Indicator" class="Bool (strict)"("BoolText.Text"="Measuring\nTransport") -> ()  [unwired: 2 in, 2 out]
            n167 = Concatenate Strings(w244, w243) -> (w242:string)
            n168 = Equal?(x=w229, y=w230) -> (x = y?=w238:bool)
            n169 = Decimal String To Number(string=w234) -> (number=w237:i32)  [unwired: 2 in, 1 out]
            n170 = call <vilib>:"Check if File or Folder Exists.vi"("path"=w222) -> ("file or folder exists?"=w224:bool, "dup path"=w223:path)  [unwired: 8 in, 1 out]
            n171 = case shown="False" w224 {
              tunnel: w223 -> [w258 w259]
              tunnel: [w257 w259] -> w221
              frame False {
                n172 = Create Folder(path (use dialog)=w258) -> (created path=w257:path)  [unwired: 2 in, 2 out]
              }
              frame True {
              }
            }
            n173 = Decimal String To Number(string=w230) -> (number=w236:i32)  [unwired: 2 in, 1 out]
            n174 = Number To Decimal String(number=w237) -> (decimal integer string=w232:string)  [unwired: 1 in]
            n175 = Select(t=w233, s=w235, f=w232) -> (s? t:f=w231:string)
            n176 = Number To Decimal String(number=w236) -> (decimal integer string=w228:string)  [unwired: 1 in]
            n177 = Select(t=w229, s=w238, f=w228) -> (s? t:f=w227:string)
            n178 = call "Build Text2"("T"=w203, "Index"=w242, "Length"=w231, "Width"=w227) -> ("Result"=w226:string)  [unwired: 10 in, 1 out]
            n179 = Build Path(base path=w221, name or relative path=w226) -> (appended path=w239:path)
            n180 = call <vilib>:"Check if File or Folder Exists.vi"("path"=w239) -> ("file or folder exists?"=w241:bool, "dup path"=w240:path)  [unwired: 8 in, 1 out]
            n181 = case shown="True" w241 {
              tunnel: w240 -> [w260 w262]
              tunnel: [w260 w261] -> w204
              frame False {
              }
              frame True {
                n182 = while {
                  tunnel: w262 -> [w264]
                  tunnel: [w263] -> w261
                  i -> [w266]
                  stop <- w267 stop-if-true
                  n183 = Path To String(path=w264) -> (string=w273:string)
                  n184 = Increment(x=w266) -> (x+1=w265:i32)
                  n185 = Number To Decimal String(number=w265) -> (decimal integer string=w271:string)  [unwired: 1 in]
                  n186 = Concatenate Strings(w273, "_", w271) -> (w270:string)
                  n187 = String To Path(string=w270) -> (path=w269:path)
                  n188 = call <vilib>:"Check if File or Folder Exists.vi"("path"=w269) -> ("file or folder exists?"=w268:bool, "dup path"=w263:path)  [unwired: 8 in, 1 out]
                  n189 = Not(x=w268) -> (.not. x?=w267:bool)
                }
              }
            }
            n190 = call "transport char run_subvi.vi"("VISA session"=w209, "Var1 sweep settings"=w252, "Var2 step settings"=w249, "integration time"=w212, "Path"=w204, "Sample Properties:"=w245) -> ("graphic display"=w210:cluster{"trace":dbl[], "trace":dbl[]}, "error?"=w248:errorcluster)  [unwired: 8 in]
            n191 = local write "error out"(w248) -> ()
            n192 = local write "TSP Path"(w204) -> ()
            n193 = local write "Transport Temp"(w210) -> ()
          }
        }
      }
      frame #6 {
        n194 = local write "Status Indicator"(FALSE) -> ()
        n195 = property on="Status Indicator" class="Bool (strict)"("BoolText.Text"="Ready") -> ()  [unwired: 2 in, 2 out]
      }
      frame #7 {
        n196 = node-c288(100) -> (w282:T8)  [unwired: 3 in]
        n197 = timed-loop {
          timing: w282 -> [_]
          timing-out: [_] -> w281
          tunnel: w277 -> [w293]
          tunnel: w276 -> [w292]
          tunnel: ["Stop \nCountdown"] -> _
          i -> [w298]
          stop <- w288 stop-if-true
          n198 = node-c288() -> ()  [unwired: 1 in, 1 out]
          n199 = local read "TRF Cluster"() -> (w287:T6)
          n200 = Unbundle By Name(w287) -> ("Loop Wait"=w285:dbl)
          n201 = Multiply(x=0.1, y=w298) -> (x*y=w296:dbl)
          n202 = Equal?(x=w292, y=w293) -> (x = y?=w294:bool)
          n203 = Select(t=0, s=w294, f=w285) -> (s? t:f=w290:dbl)
          n204 = Subtract(x=w290, y=w296) -> (x-y=w284:dbl)
          n205 = Less Or Equal To 0?(x=w284) -> (x <= 0?=w289:bool)
          n206 = Or(x=w289, y="Stop \nCountdown") -> (x .or. y?=w288:bool)
          n207 = Bundle("Loop Wait"=w285, w284) -> (w286:cluster{"Loop Wait":dbl, dbl})  [unwired: 1 in]
          n208 = property on="Status Indicator" class="Bool (strict)"("BoolText.Text"="Waiting...") -> ()  [unwired: 2 in, 2 out]
          n209 = local write "Wait Cluster"(w286) -> ()
          n210 = node-c288() -> ()  [unwired: 1 in, 1 out]
        }
        n211 = node-c288(w281) -> (w278:errorcluster)
        n212 = property on="Status Indicator" class="Bool (strict)"(error in=w278, "BoolText.Text"="Ready") -> ()  [unwired: 1 in, 2 out]
      }
      frame #8 {
        n213 = Bundle("Transfer Temp"="Transfer Temp", "Transport Temp"="Transport Temp") -> (w308:T18)  [unwired: 1 in]
        n214 = local write "Graph Cluster"(w308) -> ()
      }
    }
    n215 = local write "VISA resource name out"(w10) -> ()
  }
